vi "AddMessage.vi"() -> (0 "字符串":string)   [LabVIEW 2012]
panel:
  in  "显示模式":enum32{"ASCII", "HEX"}(radio)
  in  "确定按钮":bool
  in  "需要附加的字符":string
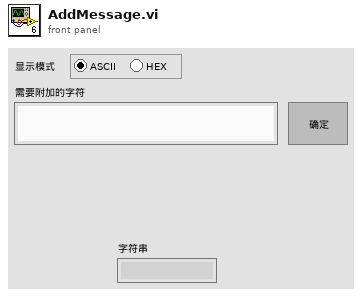
[diagram p1: front panel]
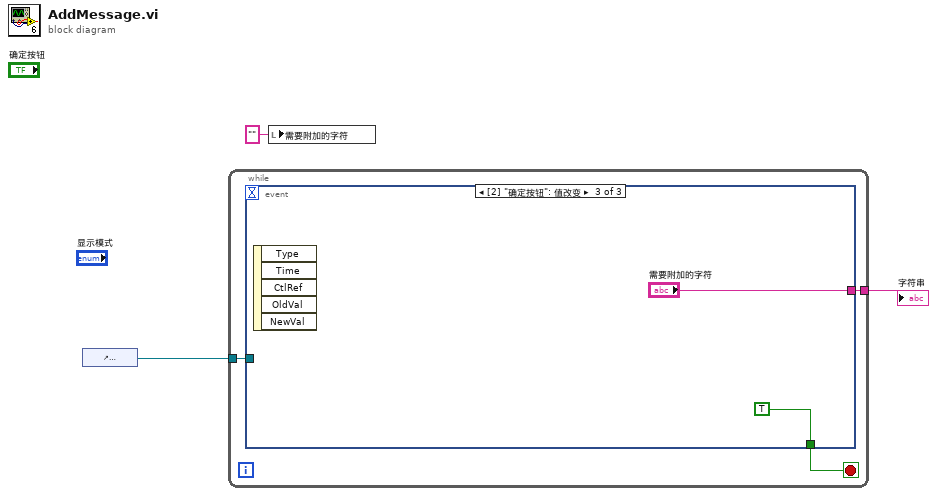
[diagram p0: block diagram]
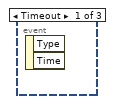
[diagram p2: hidden frame]
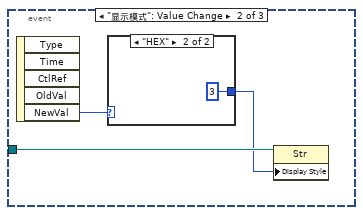
[diagram p3: hidden frame]
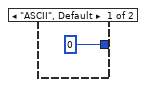
[diagram p4: hidden frame]
diagram:
  n1 = control-ref of="需要附加的字符"() -> (w3:refnum<vi>)
  n2 = while {
    tunnel: w3 -> [w6]
    tunnel: [w4] -> w2
    stop <- w5 stop-if-true
    n3 = event shown="[2] \"确定按钮\": 值改变" {
      selector: _ -> [_ _ _]
      dyn-events: _ -> [_ _ _]
      timeout: _ -> [_ _ _]
      tunnel: w6 -> [_ w9 _]
      tunnel: [_ _ TRUE] -> w5
      tunnel: [_ _ "需要附加的字符"] -> w4
      event Timeout {
        n4 = event-data() -> ()  [unwired: 1 in, 2 out]
      }
      event "显示模式": Value Change {
        n5 = event-data() -> ("NewVal"=w8:enum32{"ASCII", "HEX"})  [unwired: 1 in, 4 out]
        n6 = case shown="\"HEX\"" w8 {
          tunnel: [0 3] -> w7
          frame "ASCII", Default {
          }
          frame "HEX" {
          }
        }
        n7 = property class="Str"(reference=w9, "Display Style"=w7) -> ()  [unwired: 1 in, 2 out]
      }
      event "确定按钮": Value Change {
        n8 = event-data() -> ()  [unwired: 1 in, 5 out]
      }
    }
  }
  "字符串" <- w2
  n9 = local write "需要附加的字符"("" ("需要附加的字符")) -> ()
